vi "NT4150_Write_Integer.vi"(4 "options":T1={"Send All"=FALSE, "Keep Duplicates"=FALSE, "rate (hz)"=10}, 6 "timestamp":u64, 8 "error in":errorcluster, 9 "value":i64, 11 "name":string="Integer") -> (0 "error out":errorcluster)   [LabVIEW 2023]
doc: "Update the numeric integer to the named topic."
uses:
  <vilib>/Rock Robotics/Network Tables/NT PublishOptions.ctl
  <vilib>/Rock Robotics/Network Tables/NT Datatype.ctl
panel:
  in  "description":string="int"
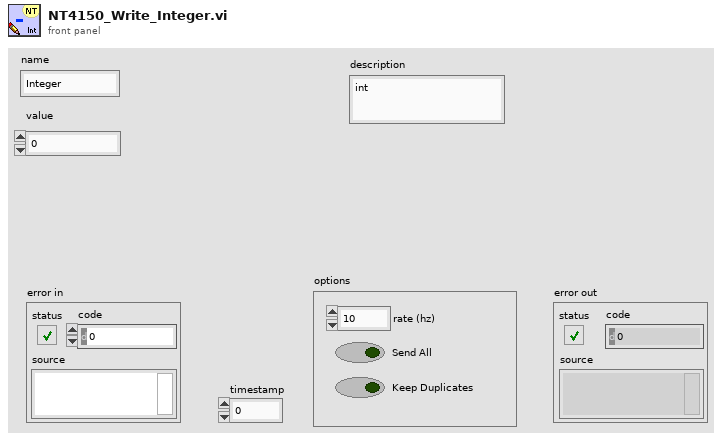
[diagram p1: front panel]
types:
  T1 = typedef "NT PublishOptions.ctl" = cluster{"Send All":bool, "Keep Duplicates":bool, "rate (hz)":u64}
  T2 = typedef "NT Datatype.ctl" = u32
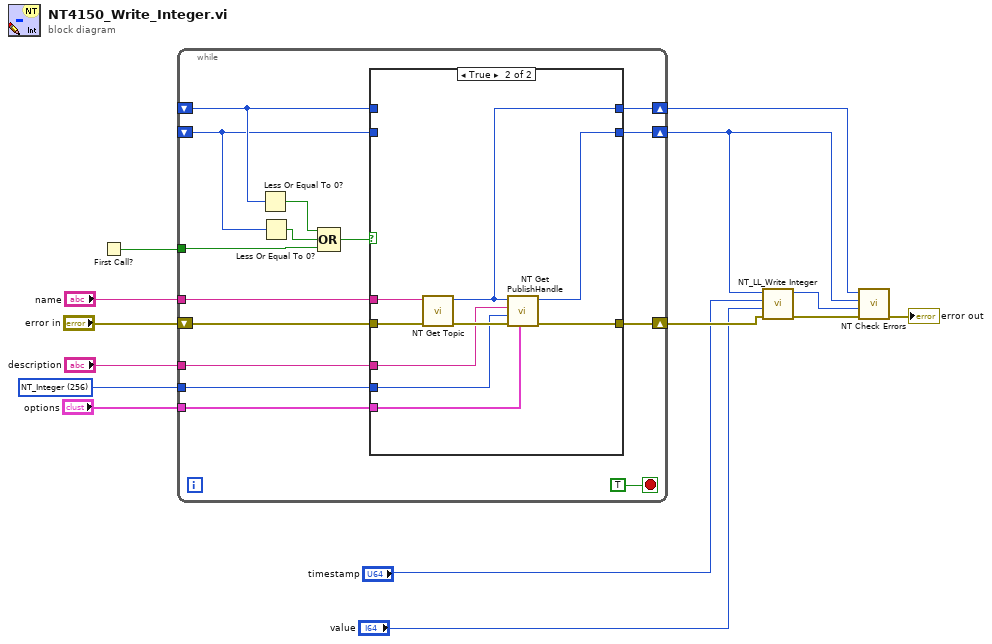
[diagram p0: block diagram]
diagram:
  w12 = T2 256 items=["NT_Unassigned"=0, "NT_Boolean"=1, "NT_Double"=2, "NT_String"=4, "NT_Raw"=8, "NT_BooleanArray"=16, "NT_DoubleArray"=32, "NT_StringArray"=64, "NT_RPC"=128, "NT_Integer"=256, "NT_Float"=512, "NT_IntegerArray"=1024, "NT_FloatArray"=2048] ("NT_Type")
  n1 = First Call?() -> (First Call?: T/F=w1:bool)
  n2 = while {
    tunnel: "name" -> [w28]
    tunnel: w12 -> [w27]
    tunnel: "description" -> [w26]
    tunnel: "options" -> [w25]
    shift-right: [w23] -> w7
    shift-left: "error in" -> [w29]
    shift-right: [w24] -> w8
    shift-left: _ -> [w16]
    shift-right: [w22] -> w4
    shift-left: _ -> [w15]
    tunnel: w1 -> [w18]
    stop <- TRUE stop-if-true
    n3 = Less Or Equal To 0?(x=w16) -> (x <= 0?=w19:bool)
    n4 = Less Or Equal To 0?(x=w15) -> (x <= 0?=w20:bool)
    n5 = Compound Arithmetic op=OR(w19, w20, w18) -> (w17:bool)
    n6 = case shown="True" w17 {
      tunnel: w29 -> [w30 w41]
      tunnel: w28 -> [_ w40]
      tunnel: w27 -> [_ w38]
      tunnel: w26 -> [_ w37]
      tunnel: w25 -> [_ w36]
      tunnel: [w32 w35] -> w24
      tunnel: [w30 w34] -> w23
      tunnel: [w31 w33] -> w22
      tunnel: w16 -> [w32 _]
      tunnel: w15 -> [w31 _]
      frame False {
      }
      frame True {
        n7 = call <vilib>:"NT Get Topic.vi"("error in (no error)"=w41, "name"=w40) -> ("error out"=w39:errorcluster, "topicHandle"=w35:u32)  [unwired: 8 in]
        n8 = call <vilib>:"NT Get PublishHandle.vi"("options"=w36, "error in (no error)"=w39, "NT_Type"=w38, "description"=w37, "topicHandle"=w35) -> ("error out"=w34:errorcluster, "publishHandle"=w33:u32)  [unwired: 5 in]
      }
    }
  }
  n9 = call <vilib>:"NT_LL_Write Integer.vi"("error in (no error)"=w7, "value"="value", "timestamp"="timestamp", "publishHandle"=w4) -> ("error out"=w6:errorcluster, "success"=w5:u32)  [unwired: 6 in]
  n10 = call <vilib>:"NT Check Errors.vi"("error in (no error)"=w6, "success"=w5, "pubSubHandle"=w4, "topicHandle"=w8) -> ("error out"=→"error out":errorcluster)  [unwired: 7 in]
